vi "SDSU_Memory.vi.bak.vi"(0 "refnum":i32, 1 "Database RefNum in":T1, 5 "Command In":string, 7 "physical unit":string, 11 "error in (no error)":errorcluster) -> (4 "refnum out":i32, 6 "message":string, 8 "Read Value":i32, 15 "error out":errorcluster)   [LabVIEW 2016]
doc: "This VI passes the addressing information in the instrument decriptor to the Instr Open VI and returns the instrument ID. You can optionally reset the instrument by setting the front panel reset control. You must run this VI before using any of the instrument driver VIs for this instrument."
uses:
  DBSHAND/private/vis/DatabaseHand_RefNum.ctl
  DBSHAND/private/vis/DatabaseHand_Element_Set(string).vi
  SDSU_GBLVariables.vi
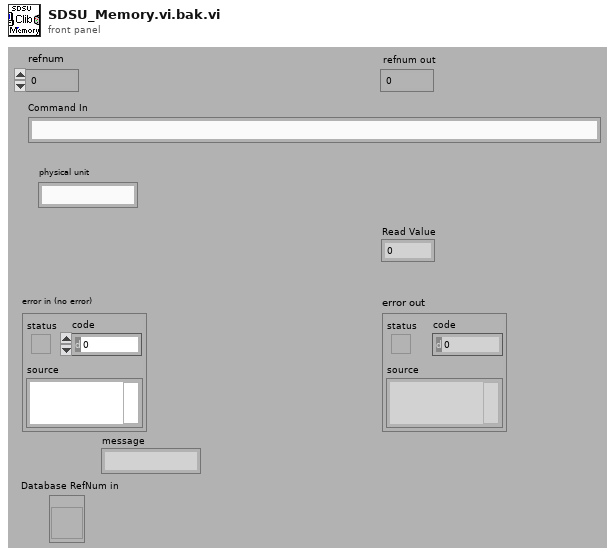
[diagram p1: front panel]
types:
  T1 = typedef "DatabaseHand_RefNum.ctl" = refnum<vi>
  T2 = enum16{"set all", "set", "get all", "get list", "get"}
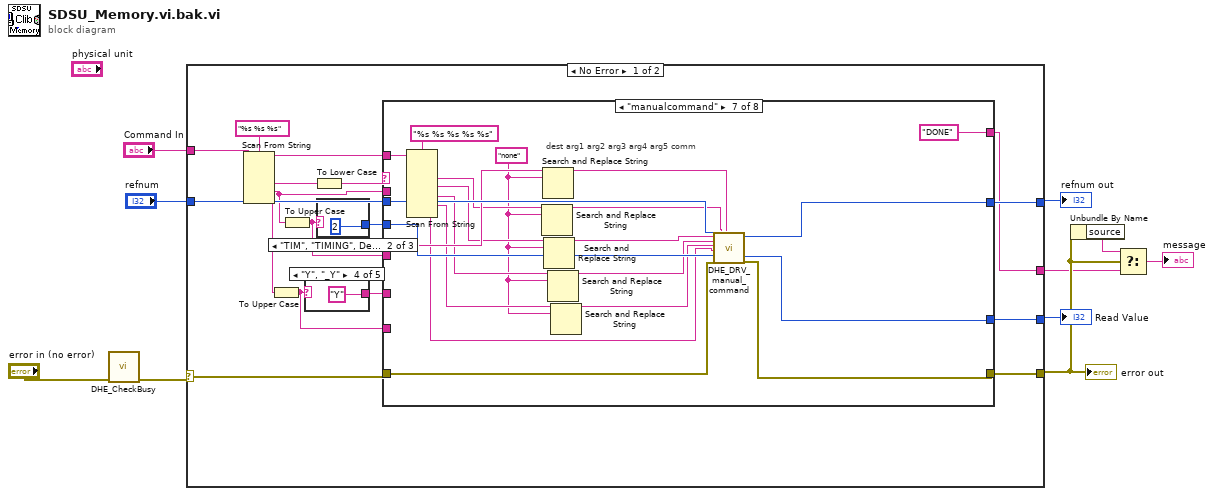
[diagram p0: block diagram]
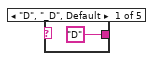
[diagram p2: hidden frame]
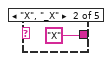
[diagram p3: hidden frame]
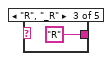
[diagram p4: hidden frame]
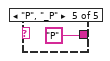
[diagram p5: hidden frame]
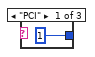
[diagram p6: hidden frame]
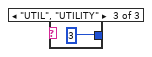
[diagram p7: hidden frame]
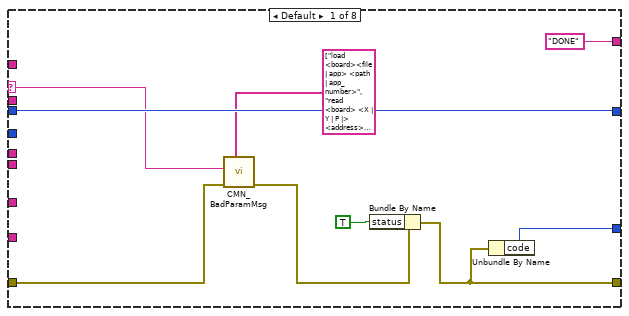
[diagram p8: hidden frame]
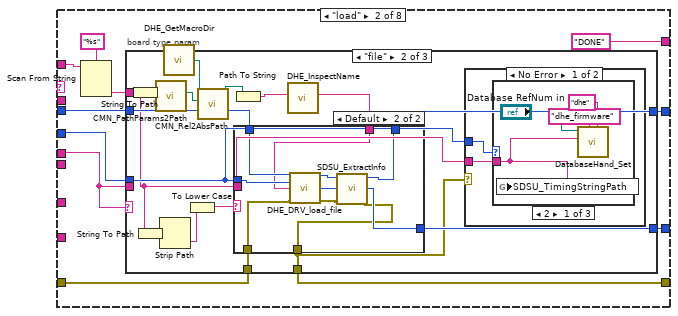
[diagram p9: hidden frame]
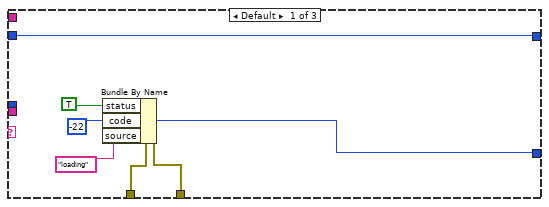
[diagram p10: hidden frame]
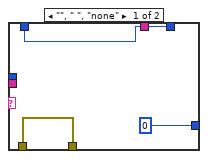
[diagram p11: hidden frame]
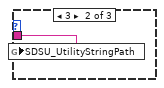
[diagram p12: hidden frame]
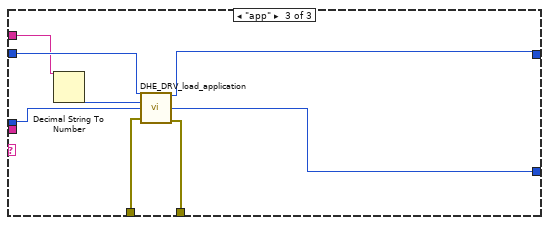
[diagram p15: hidden frame]
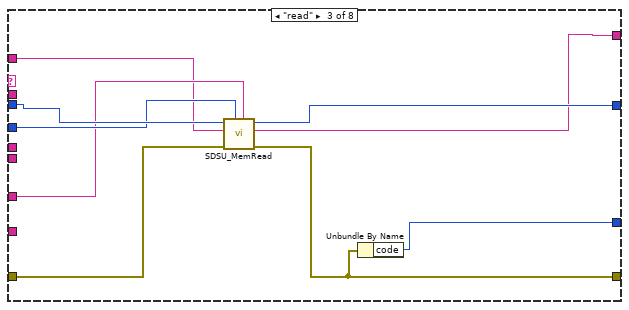
[diagram p16: hidden frame]
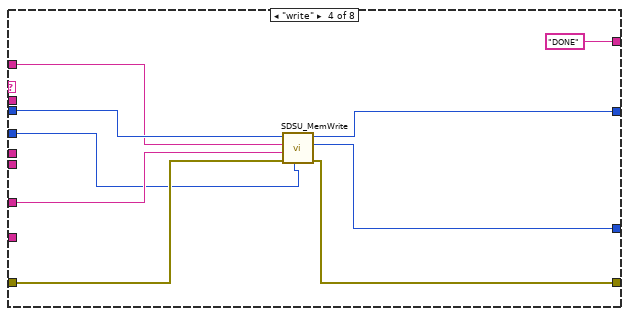
[diagram p17: hidden frame]
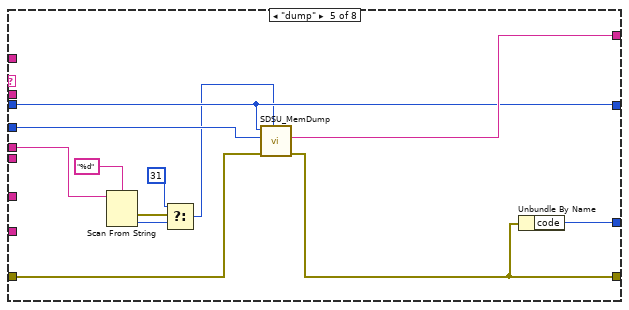
[diagram p18: hidden frame]
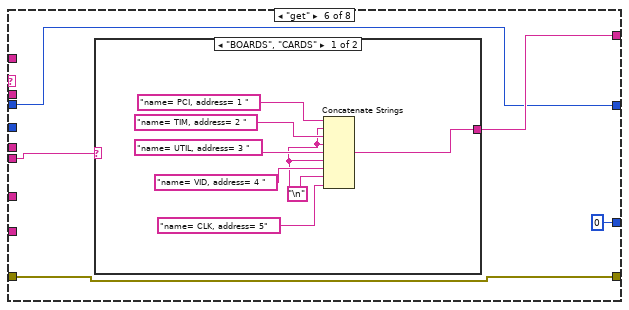
[diagram p19: hidden frame]
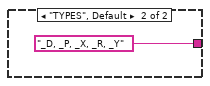
[diagram p20: hidden frame]
diagram:
  n1 = call "DHE_CheckBusy.vi"("error in (no error)"="error in (no error)") -> ("error out"=w1:errorcluster)  [unwired: 2 in, 8 out]
  n2 = case shown="No Error" w1 {
    selector: w1 -> [w23 w200]
    tunnel: [w27 w200] -> w5
    tunnel: "refnum" -> [w26 w201]
    tunnel: [w25 w201] -> w9
    tunnel: "Command In" -> [w22 _]
    tunnel: [w24 w199] -> w7
    tunnel: [w15 "ERR" ("f")] -> w2
    frame No Error {
      n3 = Scan From String(format string="%s %s %s" ("Format String"), input string=w22) -> (remaining string=w16:string, output 1=w20:string, output 2=w11:string, output 3=w13:string)  [unwired: 2 in, 5 out]
      n4 = To Upper Case(1:w13) -> (0:w12:string)
      n5 = To Upper Case(1:w11) -> (0:w14:string)
      n6 = case shown="\"Y\", \"_Y\"" w12 {
        tunnel: ["D" "X" "R" "Y" "P"] -> w19
        frame "D", "_D", Default {
        }
        frame "X", "_X" {
        }
        frame "R", "_R" {
        }
        frame "Y", "_Y" {
        }
        frame "P", "_P" {
        }
      }
      n7 = To Lower Case(string=w20) -> (all lower case string=w17:string)
      n8 = case shown="\"TIM\", \"TIMING\", Default" w14 {
        tunnel: [i16 1 i16 2 i16 3] -> w18
        frame "PCI" {
        }
        frame "TIM", "TIMING", Default {
        }
        frame "UTIL", "UTILITY" {
        }
      }
      n9 = case shown="\"manualcommand\"" w17 {
        selector: w17 -> [w42 _ _ _ _ _ _ _]
        tunnel: w23 -> [w43 w53 w110 w120 w134 w135 w164 w177]
        tunnel: [w38 w52 w106 w119 w131 w135 w163 w177] -> w27
        tunnel: w26 -> [w44 w55 w113 w121 w132 w137 w166 w171]
        tunnel: [w44 w54 w112 w118 w132 w137 w165 w171] -> w25
        tunnel: w19 -> [_ _ w108 w115 _ _ _ _]
        tunnel: [w41 w51 w105 w117 w130 0 ("error_code") w162 0 ("error_code")] -> w24
        tunnel: w13 -> [_ w49 _ _ w128 _ w160 w170]
        tunnel: w18 -> [_ w50 w109 w114 w129 _ w161 _]
        tunnel: w16 -> [_ w48 w107 w116 _ _ w168 w169]
        tunnel: ["DONE" ("f") "DONE" ("f") w111 "DONE" ("f") w133 w138 "DONE" ("f") w174] -> w15
        tunnel: w14 -> [_ _ _ _ _ w139 _ w176]
        tunnel: w12 -> [_ _ _ _ _ _ _ w173]
        tunnel: w11 -> [_ _ _ _ _ _ _ w172]
        frame Default {
          n10 = call "CMN_BadParamMsg.vi"("valid params"=string[] ["load  <board><file  | app> <path | app_number>", "read  <board> <X | Y | P |> <address>", "write <board> <X | Y | P> <address> <value>", "manualcommand <tim | util | pci> <arg1 | none> <arg2 | none> ...<arg5 | none> <command>"], "error in (no error)"=w43, "parameter"=w42) -> ("error out"=w39:errorcluster)  [unwired: 1 in, 7 out]
          n11 = Bundle By Name(cluster=w39, "status"=TRUE) -> (w38:errorcluster)
          n12 = Unbundle By Name(w38) -> ("code"=w41:i32)
        }
        frame "load" {
          # "board type param"
          n13 = Scan From String(format string="%s" ("Format String"), input string=w48) -> (output 1=w46:string)  [unwired: 2 in, 4 out]
          n14 = case shown="\"file\"" w49 {
            tunnel: w55 -> [w61 w77 w102]
            tunnel: [w61 w74 w101] -> w54
            tunnel: w53 -> [w60 w76 w104]
            tunnel: [w59 w71 w103] -> w52
            tunnel: [w56 w75 w97] -> w51
            tunnel: w50 -> [_ w73 w98]
            tunnel: w49 -> [_ _ _]
            tunnel: w46 -> [_ w64 w100]
            frame Default {
              w56 = -22
              n15 = Bundle By Name(cluster=w60, "status"=TRUE, "code"=w56, "source"="loading") -> (w59:errorcluster)
            }
            frame "file" {
              n16 = String To Path(string=w64) -> (path=w66:path)
              n17 = String To Path(string=w64) -> (path=w63:path)
              n18 = call "CMN_PathParams2Path.vi"("Path In"=w66) -> ("Path out"=w67:path)  [unwired: 2 in, 8 out]
              n19 = Strip Path(path=w63) -> (name=w62:string)  [unwired: 1 out]
              n20 = call "DHE_GetMacroDir.vi"() -> ("DHE_MacroDir"=w68:path)  [unwired: 9 out]
              n21 = To Lower Case(string=w62) -> (all lower case string=w72:string)
              n22 = call "CMN_Rel2AbsPath.vi"("test path"=w67, "absolute path"=w68) -> ("output path"=w69:path)  [unwired: 1 in, 8 out]
              n23 = Path To String(path=w69) -> (string=w70:string)
              n24 = call "DHE_InspectName.vi"("name in"=w70) -> ("name out"=w65:string)  [unwired: 10 out]
              n25 = case shown="Default" w72 {
                tunnel: w77 -> [w79 w89]
                tunnel: w76 -> [w80 w88]
                tunnel: [0 ("return value") w87] -> w75
                tunnel: [w79 w84] -> w74
                tunnel: w73 -> [_ w83]
                tunnel: w64 -> [_ _]
                tunnel: [w80 w82] -> w71
                tunnel: w65 -> [_ w81]
                frame "", " ", "none" {
                }
                frame Default {
                  n26 = call "DHE_DRV_load_file.vi"("fd"=w89, "dest"=w83, "filename"=w81, "error in (no error)"=w88) -> ("fd out"=w86:i32, "return value"=w87:i32, "error out"=w85:errorcluster)  [unwired: 9 out]
                  n27 = call "SDSU_ExtractInfo.vi"("error in (no error)"=w85, "refnum"=w86) -> ("error out"=w82:errorcluster, "refnum out"=w84:i32)  [unwired: 8 out]
                }
              }
              n28 = case shown="No Error" w71 {
                tunnel: w73 -> [w91 _]
                tunnel: w64 -> [w90 _]
                frame No Error {
                  n29 = case shown="2" w91 {
                    tunnel: w90 -> [w92 w96 _]
                    frame 2 {
                      n30 = global write "SDSU_GBLVariables.vi" "SDSU_TimingStringPath"(w92) -> ()
                      n31 = call-poly "DatabaseHand_Set.vi"("group"="dhe", "name"="dhe_firmware", "value"=w92, "Database RefNum in"="Database RefNum in") -> ()  [unwired: 4 in, 4 out]
                    }
                    frame 3 {
                      n32 = global write "SDSU_GBLVariables.vi" "SDSU_UtilityStringPath"(w96) -> ()
                    }
                    frame 1, Default {
                    }
                  }
                }
                frame Error {
                }
              }
            }
            frame "app" {
              n33 = Decimal String To Number(string=w100) -> (number=w99:i32)  [unwired: 3 out]
              n34 = call "DHE_DRV_load_application.vi"("fd"=w102, "app"=w99, "dest"=w98, "error in (no error)"=w104) -> ("fd out"=w101:i32, "return value"=w97:i32, "error out"=w103:errorcluster)  [unwired: 9 out]
            }
          }
        }
        frame "read" {
          n35 = call "SDSU_MemRead.vi"("type"=w108, "board dest"=w109, "error in (no error)"=w110, "memin"=w107, "fd"=w113) -> ("error out"=w106:errorcluster, "values"=w111:string, "fd out"=w112:i32)  [unwired: 4 out]
          n36 = Unbundle By Name(w106) -> ("code"=w105:i32)
        }
        frame "write" {
          n37 = call "SDSU_MemWrite.vi"("board dest"=w114, "error in (no error)"=w120, "type"=w115, "args"=w116, "fd"=w121) -> ("error out"=w119:errorcluster, "return value"=w117:i32, "fd out"=w118:i32)  [unwired: 4 out]
        }
        frame "dump" {
          n38 = Scan From String(format string="%d", input string=w128) -> (error out=w126:errorcluster, output 1=w125:i32)  [unwired: 2 in, 3 out]
          n39 = Select(t=31, s=w126, f=w125) -> (s? t:f=w124:i32)
          n40 = call "SDSU_MemDump.vi"("maxloc"=w124, "error in (no error)"=w134, "board dest"=w129, "refnum"=w132) -> ("error out"=w131:errorcluster, "mem"=w133:string)  [unwired: 1 in, 5 out]
          n41 = Unbundle By Name(w131) -> ("code"=w130:i32)
        }
        frame "get" {
          n42 = case shown="\"BOARDS\", \"CARDS\"" w139 {
            tunnel: [w143 "_D, _P, _X, _R, _Y"] -> w138
            frame "BOARDS", "CARDS" {
              w140 = "\n"
              n43 = Concatenate Strings("name= PCI, address= 1 ", w140, "name= TIM, address= 2 ", w140, "name= UTIL, address= 3 ", w140, "name= VID, address= 4 ", w140, "name= CLK, address= 5") -> (w143:string)
            }
            frame "TYPES", Default {
            }
          }
        }
        frame "manualcommand" {
          w155 = "none" ("search string")
          # "dest arg1 arg2 arg3 arg4 arg5 comm"
          n44 = Scan From String(format string="%s %s %s %s %s" ("Format String"), input string=w168) -> (output 1=w159:string, output 2=w158:string, output 3=w157:string, output 4=w156:string, output 5=w149:string)  [unwired: 2 in, 8 out]
          n45 = Search and Replace String(input string=w159, search string=w155) -> (result string=w153:string)  [unwired: 1 in, 8 out]
          n46 = Search and Replace String(input string=w160, search string=w155) -> (result string=w154:string)  [unwired: 1 in, 8 out]
          n47 = Search and Replace String(input string=w158, search string=w155) -> (result string=w152:string)  [unwired: 1 in, 8 out]
          n48 = Search and Replace String(input string=w157, search string=w155) -> (result string=w151:string)  [unwired: 1 in, 8 out]
          n49 = Search and Replace String(input string=w156, search string=w155) -> (result string=w150:string)  [unwired: 1 in, 8 out]
          n50 = call "DHE_DRV_manual_command.vi"("arg3"=w152, "arg4"=w151, "arg5"=w150, "command"=w149, "short board_dest"=w161, "error in (no error)"=w164, "arg2"=w153, "arg1"=w154, "fd"=w166) -> ("fd"=w165:i32, "error_code"=w162:i32, "error out"=w163:errorcluster)  [unwired: 8 out]
        }
        frame "clk", "clock", "mux" {
          n51 = case shown="\"GET\"" w176 {
            tunnel: ["ERROR unknow command to mux" ("f") w182 w186 w196] -> w174
            tunnel: w173 -> [_ _ w187 w195]
            tunnel: w172 -> [_ _ w185 _]
            tunnel: w171 -> [_ w184 _ _]
            tunnel: w170 -> [_ w181 _ _]
            tunnel: w169 -> [_ w180 _ w194]
            frame Default {
            }
            frame "SET" {
              n52 = Concatenate Strings(w181, w180) -> (w179:string)
              n53 = call "SDSU_ReadMux.vi"("fd"=w184, "argument"=w179, "action"=T2."set") -> ("response"=w182:string)  [unwired: 2 in, 6 out]
            }
            frame "GET" {
              n54 = case shown="Default" w187 {
                selector: w187 -> [w188 _]
                tunnel: [w189 w191] -> w186
                tunnel: w185 -> [_ _]
                frame Default {
                  n55 = call "SDSU_ReadMux.vi"("argument"=w188, "action"=T2."get") -> ("response"=w189:string)  [unwired: 3 in, 6 out]
                }
                frame "LIST" {
                  n56 = call "SDSU_ReadMux.vi"("action"=T2."get list") -> ("response"=w191:string)  [unwired: 4 in, 6 out]
                }
              }
            }
            frame "GETALL" {
              n57 = Concatenate Strings(w195, w194) -> (w193:string)
              n58 = call "SDSU_ReadMux.vi"("argument"=w193, "action"=T2."get all") -> ("response"=w196:string)  [unwired: 3 in, 6 out]
            }
          }
        }
      }
    }
    frame Error {
      n59 = Unbundle By Name(w200) -> ("code"=w199:i32)
    }
  }
  "error out" <- w5
  "refnum out" <- w9
  "Read Value" <- w7
  n60 = Unbundle By Name(w5) -> ("source"=w4:string)
  n61 = Select(t=w4, s=w5, f=w2) -> (s? t:f=→"message":string)
